vi "KE622x -- Set Questionable Event Enable Reg State.vi"(0 "VISA Resource In":refnum<visa-resource-name>, 1 "Error Query (T)?":bool=TRUE, 7 "KE622x Questionable Event Enabled Reg":T1, 11 "error in (no error)":errorcluster) -> (4 "VISA Resource Out (dupl)":refnum<visa-resource-name>, 15 "error out":errorcluster)   [LabVIEW 2009, in "Keithley 622x.lvlib"]
doc: "Sets the bits in the 'Questionable Event Enable' register of the Status Model. Note that only the used (named) bits are settable -- all other bits default to zero."
uses:
  <instrlib>/Keithley 622x LV 2009/Utility/Status Registers/Typedefs/KE622x -- Questionable Event Enable Reg State.ctl
  <instrlib>/Keithley 622x LV 2009/Keithley 622x.lvlib
panel:
  out "Reg Num (dec)":u16 format="%0d"
  out "Reg Num (binary)":u16 format="%016b"
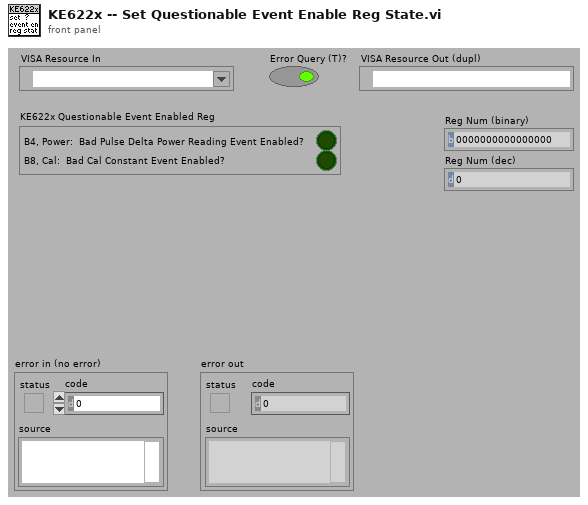
[diagram p1: front panel]
types:
  T1 = typedef "Keithley 622x.lvlib/KE622x -- Questionable Event Enable Reg State.ctl" = cluster{"B4, Power:  Bad Pulse Delta Power Reading Event Enabled?":bool, "B8, Cal:  Bad Cal Constant Event Enabled?":bool}
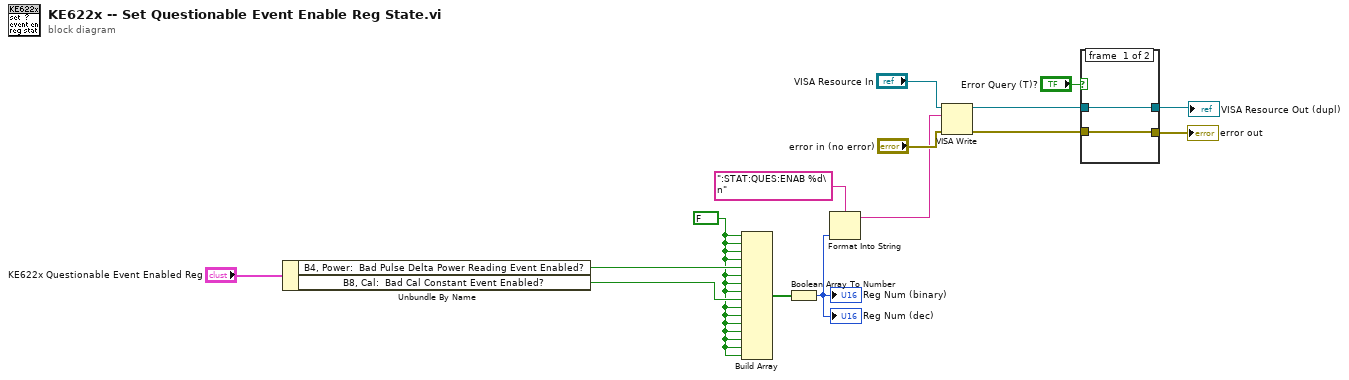
[diagram p0: block diagram]
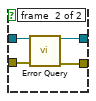
[diagram p2: hidden frame]
diagram:
  w1 = FALSE
  n1 = Unbundle By Name("KE622x Questionable Event Enabled Reg") -> ("B4, Power:  Bad Pulse Delta Power Reading Event Enabled?"=w3:bool, "B8, Cal:  Bad Cal Constant Event Enabled?"=w2:bool)
  n2 = Build Array(w1, w1, w1, w1, w3, w1, w1, w1, w2, w1, w1, w1, w1, w1, w1, w1) -> (w15:bool[])
  n3 = Boolean Array To Number(Boolean array=w15) -> (number=w12:u32)
  "Reg Num (binary)" <- w12
  "Reg Num (dec)" <- w12
  n4 = Format Into String(format string=":STAT:QUES:ENAB %d\n" ("write buffer"), w12) -> (resulting string=w10:string)  [unwired: 2 in, 1 out]
  n5 = VISA Write(VISA resource name="VISA Resource In", write buffer=w10, error in (no error)="error in (no error)") -> (VISA resource name out=w8:refnum<visa-resource-name>, error out=w9:errorcluster)  [unwired: 1 out]
  n6 = case shown="True" "Error Query (T)?" {
    tunnel: w9 -> [w16 w21]
    tunnel: w8 -> [w17 w20]
    tunnel: [w16 w19] -> w7
    tunnel: [w17 w18] -> w6
    frame #0 {
    }
    frame #1 {
      n7 = call <instrlib>:"Error Query.vi"("VISA Resource In"=w20, "error in (no error)"=w21) -> ("VISA Resource Out (dupl)"=w18:refnum<visa-resource-name>, "error out"=w19:errorcluster)  [unwired: 10 in, 2 out]
    }
  }
  "VISA Resource Out (dupl)" <- w6
  "error out" <- w7
